vi "TestDLL.vi"() -> ()   [LabVIEW 2020]
uses:
  LVT32.dll
panel:
  out "v_Write":T1
  out "v_Access":T1
  out "v_Creation":T1
  out "f_Result 2":i32
  out "v_CalChecksum":u16 format="%04x"
  out "v_RefChecksum":u16 format="%04x"
  out "f_Result":i32
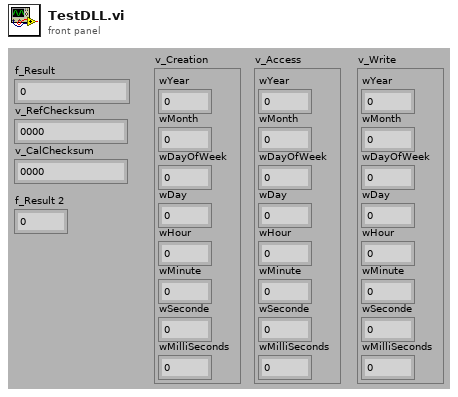
[diagram p1: front panel]
types:
  T1 = cluster{"wYear":u16, "wMonth":u16, "wDayOfWeek":u16, "wDay":u16, "wHour":u16, "wMinute":u16, "wSeconde":u16, "wMilliSeconds":u16}
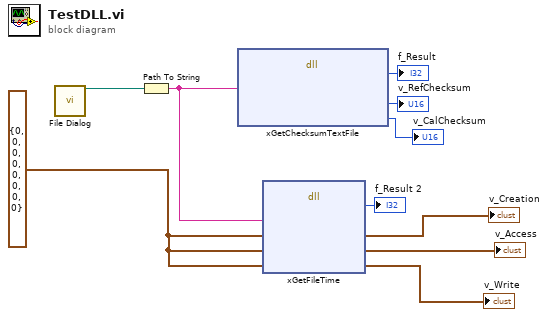
[diagram p0: block diagram]
diagram:
  w4 = T1 {"wYear"=0, "wMonth"=0, "wDayOfWeek"=0, "wDay"=0, "wHour"=0, "wMinute"=0, "wSeconde"=0, "wMilliSeconds"=0} ("System")
  n1 = call "File Dialog"() -> ("selected path"=w7:path)  [unwired: 12 in, 3 out]
  n2 = Path To String(path=w7) -> (string=w6:string)
  n3 = dll-call lib="C:/Factory/FactoryGenericTools/Dll/LVT32.dll" fn="xGetChecksumTextFile"("c_Path"=w6) -> ("f_Result"=→"f_Result":i32, "v_RefChecksum"=→"v_RefChecksum":u16, "v_CalChecksum"=→"v_CalChecksum":u16)  [unwired: 6 in, 2 out]
  n4 = dll-call lib="C:/Factory/FactoryGenericTools/Dll/LVT32.dll" fn="xGetFileTime"("c_Path"=w6, "v_Creation"=w4, "v_Access"=w4, "v_Write"=w4) -> ("f_Result"=→"f_Result 2":i32, "v_Creation"=→"v_Creation":T1, "v_Access"=→"v_Access":T1, "v_Write"=→"v_Write":T1)  [unwired: 4 in, 2 out]
